vi "sub_psk_symbol_map_gen.vi"(9 "Gray code?":bool=TRUE, 11 "M-PSK":i32=4) -> (1 "index map":u32[](array[numeric]), 3 "symbol map":cdb[](array[numeric]))   [LabVIEW 2014]
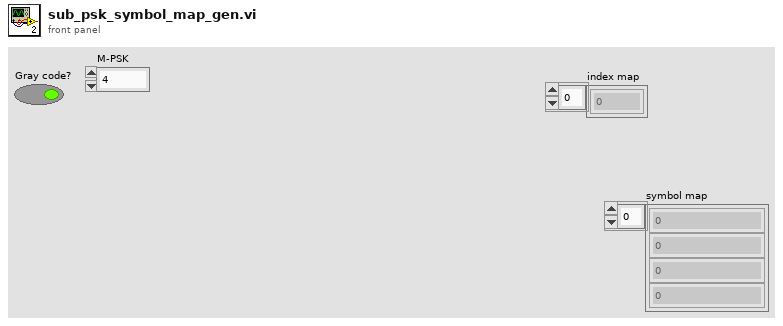
[diagram p1: front panel]
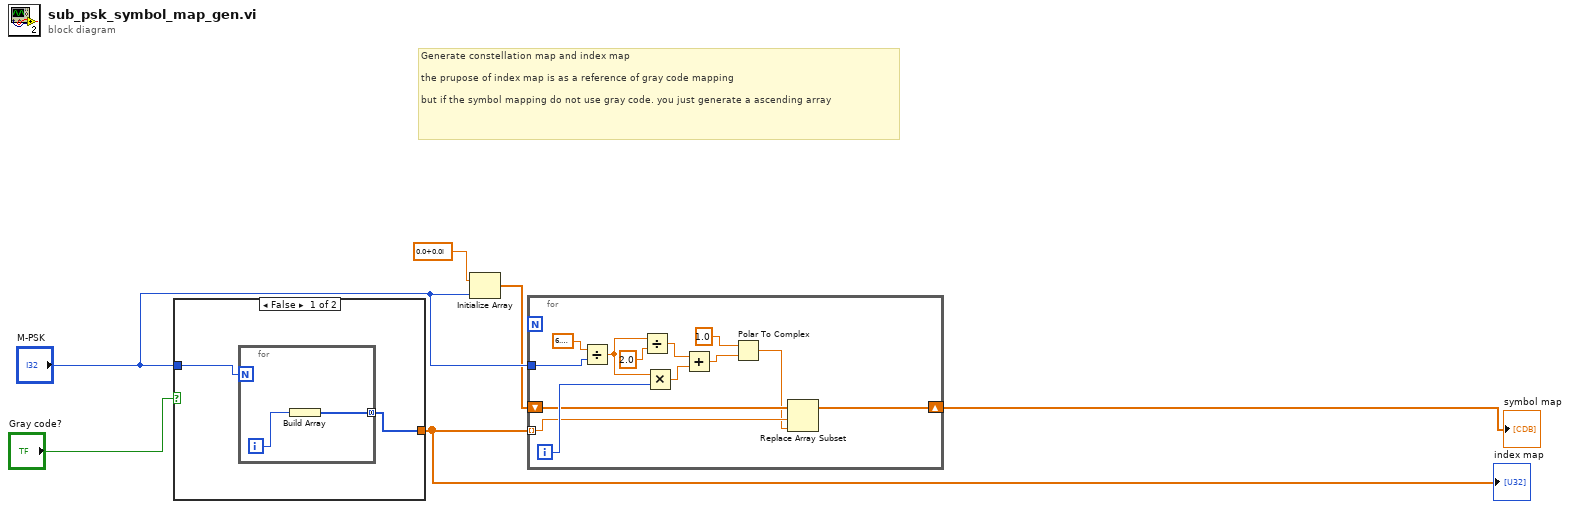
[diagram p0: block diagram]
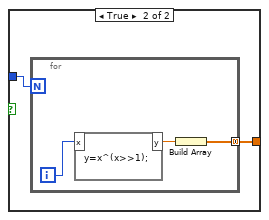
[diagram p2: hidden frame]
diagram:
  # "Generate constellation map and index map\n\nthe prupose of index map is as a reference of gray code mapping\n\nbut if the symbol mapping do not use gray code. you just generate a ascending array"
  n1 = case shown="False" "Gray code?" {
    tunnel: "M-PSK" -> [w8 w12]
    tunnel: [w7 w11] -> w5
    frame False {
      n2 = for {
        N: w8 -> [_]
        tunnel: [w9] -> w7 mode=concatenating
        i -> [w10]
        n3 = Build Array(w10) -> (w9:i32[])
      }
    }
    frame True {
      n4 = for {
        N: w12 -> [_]
        tunnel: [w13] -> w11 mode=concatenating
        i -> [w15]
        n5 = formula code="y=x^(x>>1);"("x"=w15) -> ("y"=w14:dbl)
        n6 = Build Array(w14) -> (w13:dbl[])
      }
    }
  }
  "index map" <- w5
  n7 = Initialize Array(cdb 0.0+0.0i, "M-PSK") -> (w2:cdb[])
  n8 = for {
    tunnel: w5 -> [w18] mode=indexing
    tunnel: "M-PSK" -> [w27]
    shift-right: [w16] -> w1
    shift-left: w2 -> [w19]
    i -> [w25]
    n9 = Divide(x=6.283185307179586, y=w27) -> (x/y=w24:dbl)
    n10 = Divide(x=w24, y=2.0) -> (x/y=w23:dbl)
    n11 = Multiply(x=w24, y=w25) -> (x*y=w22:dbl)
    n12 = Add(x=w23, y=w22) -> (x+y=w21:dbl)
    n13 = Polar To Complex(1:w21, 2:1.0) -> (0:w17:cdb)
    n14 = Replace Array Subset(array=w19, new element=w17, index=w18) -> (w16:cdb[])
  }
  "symbol map" <- w1
